vi "ConvertVSEnumToPath.vi"(10 "Source.Path Type":T1(ring), 11 "Path In":path) -> (3 "appended path":path)   [LabVIEW 2019, in "Configuration Tool.lvlib"]
uses:
  Configuration Tool.lvlib
  <vilib>/Utility/sysdir.llb/System Directory Type.ctl
  Global Settings.vi
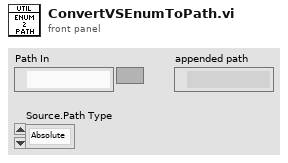
[diagram p1: front panel]
types:
  T1 = enum16{"Absolute", "To Base", "To Common Doc Dir", "To Application Data Dir"}
  T2 = typedef "System Directory Type.ctl" = i32
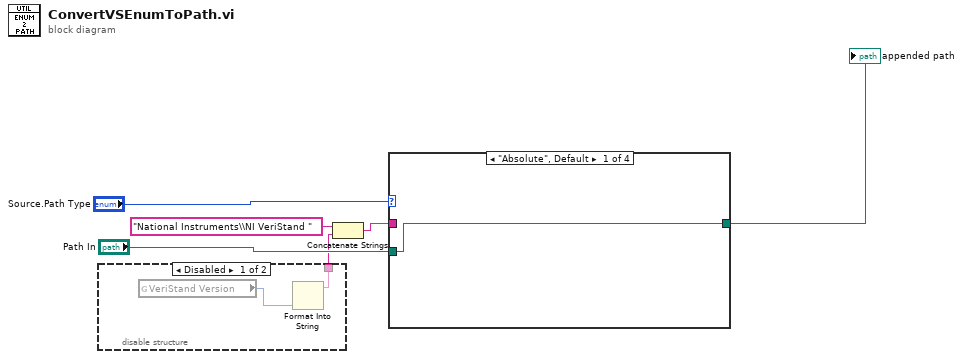
[diagram p0: block diagram]
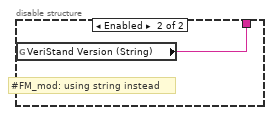
[diagram p2: hidden frame]
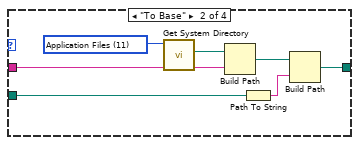
[diagram p3: hidden frame]
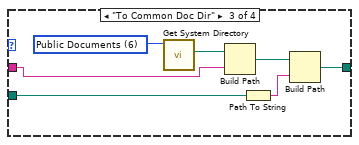
[diagram p4: hidden frame]
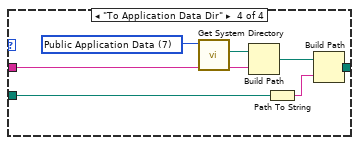
[diagram p5: hidden frame]
diagram:
  n1 = disable-structure shown="Disabled" {
    disable-tunnel: [w7 w9] -> w2
    frame Disabled {
      n2 = global read "Global Settings.vi" "VeriStand Version"() -> (w8:enum16{"2013", "2014", "2015", "2016"})
      n3 = Format Into String(w8) -> (resulting string=w7:string)  [unwired: 3 in, 1 out]
    }
    frame Enabled {
      # "#FM_mod: using string instead"
      n4 = global read "Global Settings.vi" "VeriStand Version (String)"() -> (w9:string)
    }
  }
  n5 = Concatenate Strings("National Instruments\\NI VeriStand " ("name or relative path"), w2) -> (w1:string)
  n6 = case shown="\"Absolute\", Default" "Source.Path Type" {
    tunnel: "Path In" -> [w10 w13 w20 w27]
    tunnel: [w10 w12 w19 w26] -> w6
    tunnel: w1 -> [_ w11 w18 w25]
    frame "Absolute", Default {
    }
    frame "To Base" {
      w17 = T2 11 items=["User Home"=0, "User Desktop"=1, "User Documents"=2, "User Application Data"=3, "User Preferences"=4, "User Temporary"=5, "Public Documents"=6, "Public Application Data"=7, "Public Preferences"=8, "Public Cache"=13, "System Core Libraries"=9, "System Installed Libraries"=10, "Application Files"=11, "Boot Volume Root"=12] ("system directory type")
      n7 = call <vilib>:"Get System Directory.vi"("system directory type"=w17) -> ("system directory"=w16:path)  [unwired: 10 in]
      n8 = Build Path(base path=w16, name or relative path=w11) -> (appended path=w15:path)
      n9 = Path To String(path=w13) -> (string=w14:string)
      n10 = Build Path(base path=w15, name or relative path=w14) -> (appended path=w12:path)
    }
    frame "To Common Doc Dir" {
      w24 = T2 6 items=["User Home"=0, "User Desktop"=1, "User Documents"=2, "User Application Data"=3, "User Preferences"=4, "User Temporary"=5, "Public Documents"=6, "Public Application Data"=7, "Public Preferences"=8, "Public Cache"=13, "System Core Libraries"=9, "System Installed Libraries"=10, "Application Files"=11, "Boot Volume Root"=12] ("system directory type")
      n11 = call <vilib>:"Get System Directory.vi"("system directory type"=w24) -> ("system directory"=w23:path)  [unwired: 10 in]
      n12 = Build Path(base path=w23, name or relative path=w18) -> (appended path=w22:path)
      n13 = Path To String(path=w20) -> (string=w21:string)
      n14 = Build Path(base path=w22, name or relative path=w21) -> (appended path=w19:path)
    }
    frame "To Application Data Dir" {
      w31 = T2 7 items=["User Home"=0, "User Desktop"=1, "User Documents"=2, "User Application Data"=3, "User Preferences"=4, "User Temporary"=5, "Public Documents"=6, "Public Application Data"=7, "Public Preferences"=8, "Public Cache"=13, "System Core Libraries"=9, "System Installed Libraries"=10, "Application Files"=11, "Boot Volume Root"=12] ("system directory type")
      n15 = call <vilib>:"Get System Directory.vi"("system directory type"=w31) -> ("system directory"=w30:path)  [unwired: 10 in]
      n16 = Build Path(base path=w30, name or relative path=w25) -> (appended path=w29:path)
      n17 = Path To String(path=w27) -> (string=w28:string)
      n18 = Build Path(base path=w29, name or relative path=w28) -> (appended path=w26:path)
    }
  }
  "appended path" <- w6
